vi "Exemple_Impute_MissingIndicator.vi"() -> ()   [LabVIEW 2020]
uses:
  Objet/6 - Datasets Transformation/6.4 - Imputation of missing values/MissingIndicator/MissingIndicator.lvclass
panel:
  in  "X":string[][](array[string])=[["nan", "1", "3"], ["4", "0", "nan"], ["8", "1", "0"]]
  in  "MissingIndicator":T1={"missing_values"="nan", "features"="missing-only", "sparse"="auto", "error_on_new"=TRUE}
  out "Data":T2
  out "error out":errorcluster caption="sortie d'erreur"
  in  "error in":errorcluster caption="entrée d'erreur"
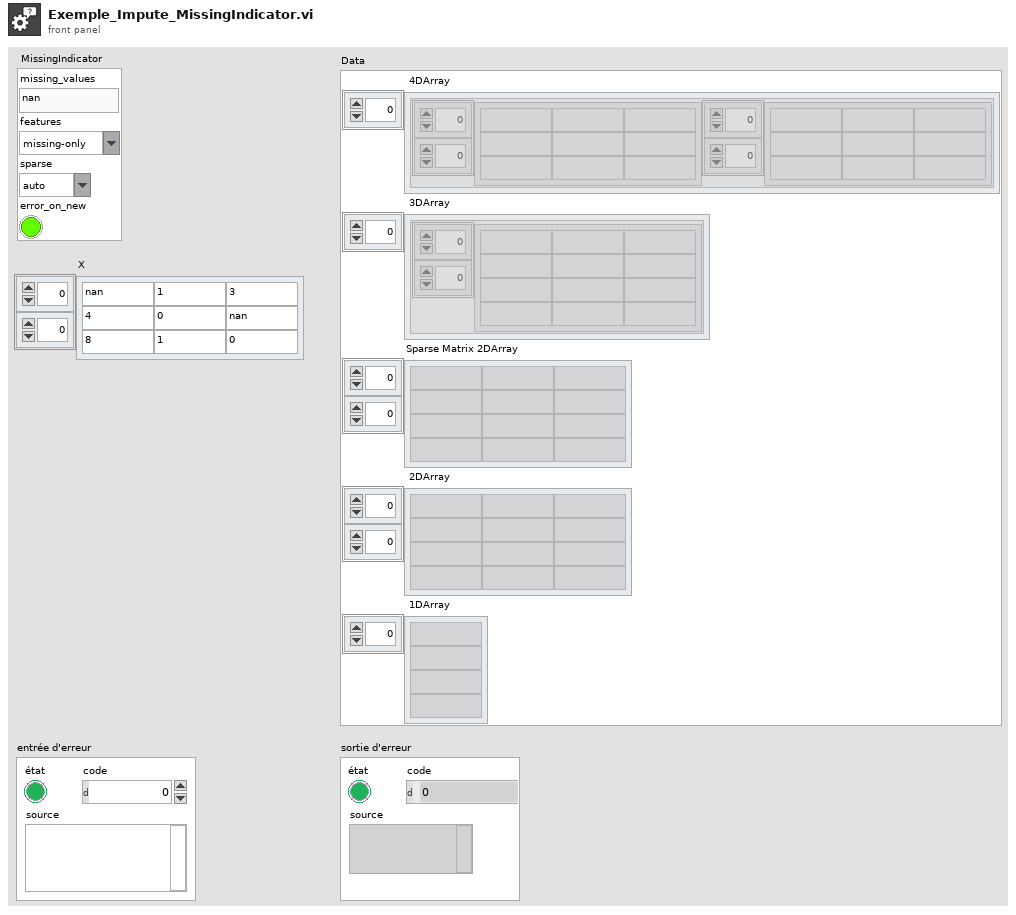
[diagram p1: front panel]
types:
  T1 = cluster{"missing_values":string, "features":string, "sparse":string, "error_on_new":bool}
  T2 = cluster{" 4DArray":cluster{"1":string[][], "2":string[][]}[], " 3DArray":cluster{"Tableau":string[][]}[], "Sparse Matrix 2DArray":string[][], " 2DArray":string[][], " 1DArray":string[]}
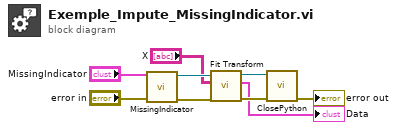
[diagram p0: block diagram]
diagram:
  n1 = call "MissingIndicator.vi"("error in"="error in", "MissingIndicator"="MissingIndicator") -> ("error out"=w6:errorcluster, "MissingIndicator.lvclass"=w9:refnum<class "MissingIndicator.lvclass">)  [unwired: 8 in]
  n2 = call-dynamic "Fit Transform.vi"("error in (no error)"=w6, "X"="X", "MissingIndicator.lvclass"=w9) -> ("error out"=w4:errorcluster, "Data"=→"Data":T2, "MissingIndicator.lvclass"=w5:refnum<class "MissingIndicator.lvclass">)  [unwired: 6 in]
  n3 = call-dynamic "ClosePython.vi"("error in (no error)"=w4, "Scikit-learn en entrée"=w5) -> ("error out"=→"error out":errorcluster)  [unwired: 8 in, 1 out]
